vi "Tap_valuation.vi"(0 "1st_Col.":i32, 1 "1st_moveLog":i32[][](array[numeric]), 3 "1st_TotalP":i32, 5 "1st_TapN":dbl, 9 "2nd_TotalP":i32, 11 "2nd_moveLog":i32[][](array[numeric]), 12 "2nd Col.":i32, 13 "2nd_TapN":dbl, 14 "start Col.":i32) -> (4 "1st or 2nd":enum16{"1>2", "1=2", "1<2"}(ring), 6 "Out_TotalP":i32, 8 "Out_TapN":dbl, 10 "OutPut_moveLog":i32[][](array[numeric]), 15 "Out_ Col.":i32)   [LabVIEW 2016]
panel:
  out "Result":string
  out "1stmoveN":i32
  out "2ndmoveN":i32
  # "優先順位(1:1st, 2:2nd)\n① : TapN \n      ①-1 : 1<2 → 1\n      ①-2 : 1>2 → 2\n      ①-3 : 1=2 → ②へ\n② : start Col. dev\n      ②-1 : |1-s|<|2-s|→1\n      ②-2 : |1-s|>|2-s|→2\n      ③-3 : |1-s|=|2-s|→③\n③ : TotalP\n　　　③-1 : 1≦2 →1\n      ③-2 : 1>2 → 2\n　　　③-3 : 1=2 → ④\n④: moveLogの移動少なさ\n　　　④-1 : 1≦2 →1\n      ④-2 : 1>2 → 2\n　　　④-3 : 1=2 → ④"
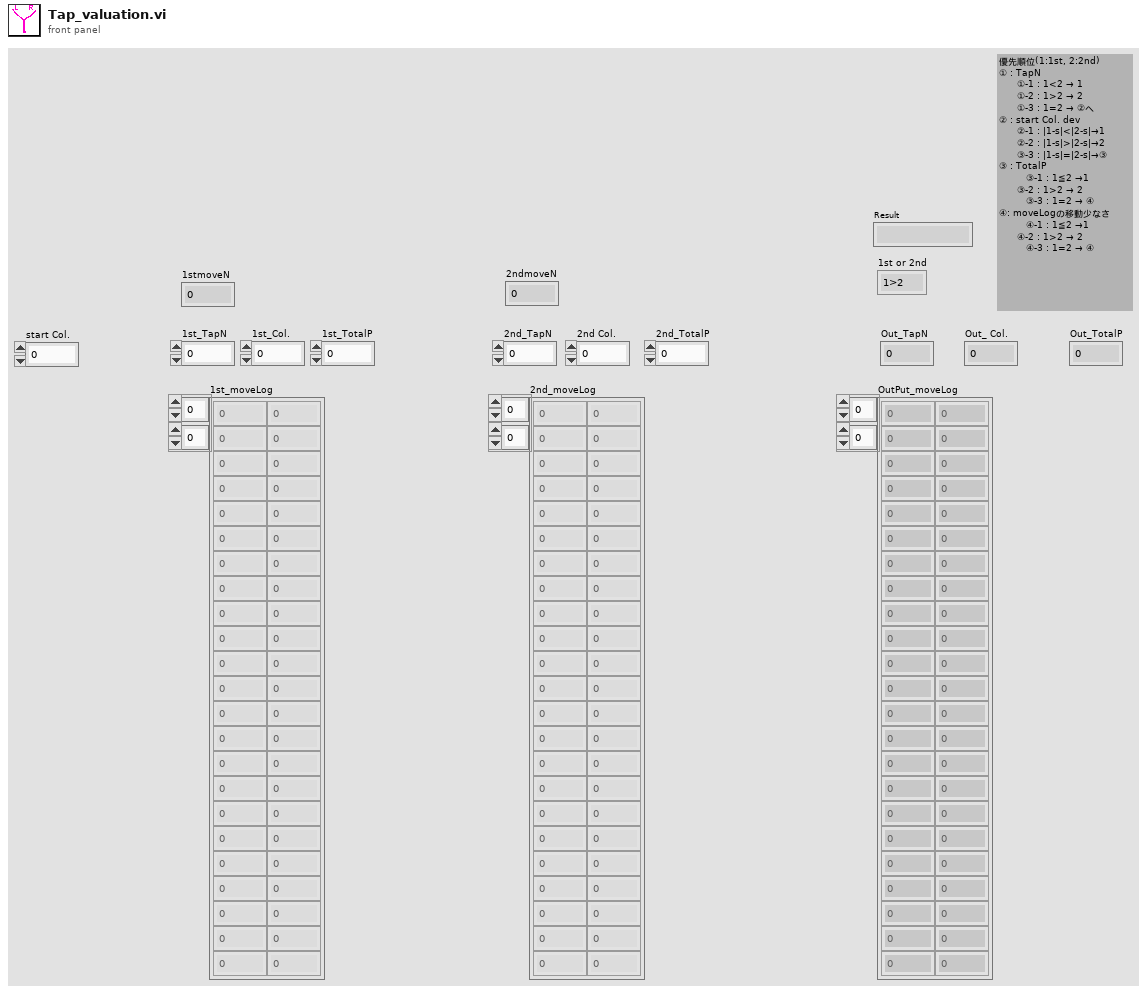
[diagram p1: front panel]
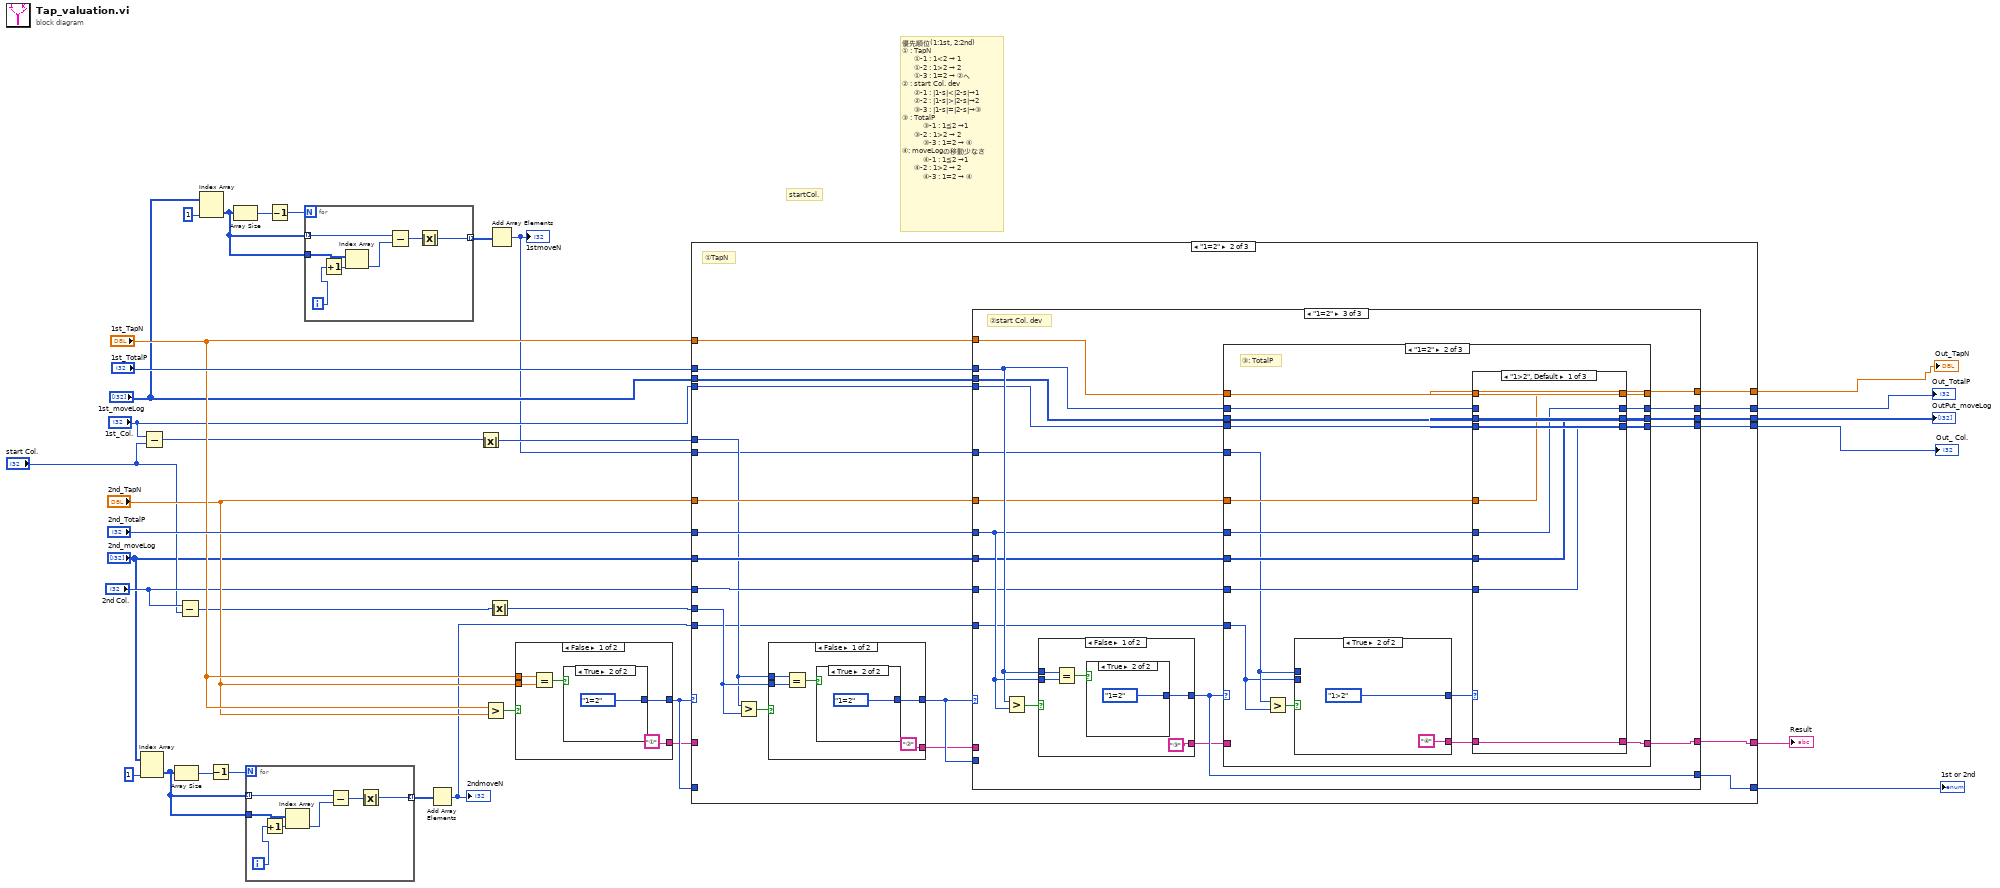
[diagram p0: block diagram]
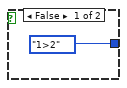
[diagram p2: hidden frame]
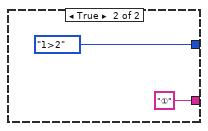
[diagram p3: hidden frame]
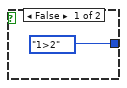
[diagram p5: hidden frame]
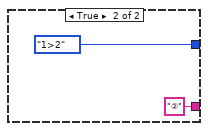
[diagram p6: hidden frame]
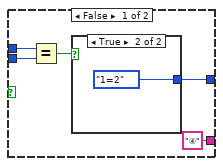
[diagram p12: hidden frame]
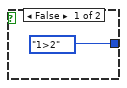
[diagram p13: hidden frame]
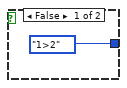
[diagram p15: hidden frame]
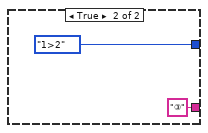
[diagram p16: hidden frame]
diagram:
  # "優先順位(1:1st, 2:2nd)\n① : TapN \n      ①-1 : 1<2 → 1\n      ①-2 : 1>2 → 2\n      ①-3 : 1=2 → ②へ\n② : start Col. dev\n      ②-1 : |1-s|<|2-s|→1\n      ②-2 : |1-s|>|2-s|→2\n      ③-3 : |1-s|=|2-s|→③\n③ : TotalP\n　　　③-1 : 1≦2 →1\n      ③-2 : 1>2 → 2\n　　　③-3 : 1=2 → ④\n④: moveLogの移動少なさ\n　　　④-1 : 1≦2 →1\n      ④-2 : 1>2 → 2\n　　　④-3 : 1=2 → ④"
  # "startCol."
  n1 = Index Array(array="2nd_moveLog", index (col)=1 ("無効な指標 （列）")) -> (element=w14:i32[])  [unwired: 1 in]
  n2 = Subtract(x="1st_Col.", y="start Col.") -> (x-y=w22:i32)
  n3 = Array Size(array=w14) -> (size(s)=w13:i32)
  n4 = Subtract(x="2nd Col.", y="start Col.") -> (x-y=w20:i32)
  n5 = Index Array(array="1st_moveLog", index (col)=1 ("無効な指標 （列）")) -> (element=w7:i32[])  [unwired: 1 in]
  n6 = Decrement(x=w13) -> (x-1=w12:i32)
  n7 = Array Size(array=w7) -> (size(s)=w8:i32)
  n8 = for {
    N: w12 -> [_]
    tunnel: w14 -> [w38] mode=indexing
    tunnel: w14 -> [w41]
    tunnel: [w35] -> w11 mode=indexing
    i -> [w39]
    n9 = Increment(x=w39) -> (x+1=w40:i32)
    n10 = Index Array(array=w41, index=w40) -> (element=w37:i32)
    n11 = Subtract(x=w38, y=w37) -> (x-y=w36:i32)
    n12 = Absolute Value(x=w36) -> (abs(x)=w35:i32)
  }
  n13 = Decrement(x=w8) -> (x-1=w9:i32)
  n14 = for {
    N: w9 -> [_]
    tunnel: w7 -> [w45] mode=indexing
    tunnel: w7 -> [w48]
    tunnel: [w42] -> w10 mode=indexing
    i -> [w46]
    n15 = Increment(x=w46) -> (x+1=w47:i32)
    n16 = Index Array(array=w48, index=w47) -> (element=w44:i32)
    n17 = Subtract(x=w45, y=w44) -> (x-y=w43:i32)
    n18 = Absolute Value(x=w43) -> (abs(x)=w42:i32)
  }
  n19 = Add Array Elements(numeric array=w11) -> (sum=w3:i32)
  "2ndmoveN" <- w3
  n20 = Absolute Value(x=w22) -> (abs(x)=w21:i32)
  n21 = Greater?(x="1st_TapN", y="2nd_TapN") -> (0:w28:bool)
  n22 = Absolute Value(x=w20) -> (abs(x)=w19:i32)
  n23 = Add Array Elements(numeric array=w10) -> (sum=w4:i32)
  "1stmoveN" <- w4
  n24 = case shown="False" w28 {
    tunnel: [w53 enum16{"1>2", "1=2", "1<2"}."1>2"] -> w18
    tunnel: "1st_TapN" -> [w52 _]
    tunnel: "2nd_TapN" -> [w51 _]
    tunnel: ["①" "①"] -> w2
    frame False {
      n25 = Equal?(x=w52, y=w51) -> (x = y?=w50:bool)
      n26 = case shown="True" w50 {
        tunnel: [enum16{"1>2", "1=2", "1<2"}."1>2" enum16{"1>2", "1=2", "1<2"}."1=2"] -> w53
        frame False {
        }
        frame True {
        }
      }
    }
    frame True {
    }
  }
  n27 = case shown="\"1=2\"" w18 {
    tunnel: "2nd_moveLog" -> [w61 w84 _]
    tunnel: "1st_moveLog" -> [_ w82 w190]
    tunnel: "2nd Col." -> [w60 w83 _]
    tunnel: "1st_Col." -> [_ w81 w188]
    tunnel: [w61 w79 w190] -> w32
    tunnel: "1st_TotalP" -> [_ w74 w189]
    tunnel: "2nd_TotalP" -> [w62 w73 _]
    tunnel: [w62 w80 w189] -> w31
    tunnel: [w60 w78 w188] -> w30
    tunnel: "2nd_TapN" -> [w63 w76 _]
    tunnel: "1st_TapN" -> [_ w75 w187]
    tunnel: [w63 w77 w187] -> w29
    tunnel: w21 -> [_ w70 _]
    tunnel: w19 -> [_ w71 _]
    tunnel: w18 -> [w59 _ w186]
    tunnel: [w59 w68 w186] -> w17
    tunnel: w4 -> [_ w67 _]
    tunnel: w3 -> [_ w66 _]
    tunnel: w2 -> [w58 _ w185]
    tunnel: [w58 w65 w185] -> w1
    frame "1>2", Default {
    }
    frame "1=2" {
      # "①TapN"
      n28 = Greater?(x=w70, y=w71) -> (0:w72:bool)
      n29 = case shown="False" w72 {
        tunnel: [w89 enum16{"1>2", "1=2", "1<2"}."1>2"] -> w69
        tunnel: w70 -> [w88 _]
        tunnel: w71 -> [w87 _]
        tunnel: ["②" "②"] -> w64
        frame False {
          n30 = Equal?(x=w88, y=w87) -> (x = y?=w86:bool)
          n31 = case shown="True" w86 {
            tunnel: [enum16{"1>2", "1=2", "1<2"}."1>2" enum16{"1>2", "1=2", "1<2"}."1=2"] -> w89
            frame False {
            }
            frame True {
            }
          }
        }
        frame True {
        }
      }
      n32 = case shown="\"1=2\"" w69 {
        tunnel: [w98 w105 w119] -> w80
        tunnel: w73 -> [w98 _ w113]
        tunnel: w84 -> [w97 _ w112]
        tunnel: [w97 w104 w118] -> w79
        tunnel: [w96 w103 w116] -> w78
        tunnel: w83 -> [w96 _ w111]
        tunnel: w74 -> [_ w105 w120]
        tunnel: w82 -> [_ w104 w117]
        tunnel: w81 -> [_ w103 w115]
        tunnel: w75 -> [_ w102 w121]
        tunnel: [w99 w102 w122] -> w77
        tunnel: w76 -> [w99 _ w114]
        tunnel: w69 -> [w95 w101 _]
        tunnel: [w95 w101 w110] -> w68
        tunnel: w67 -> [_ _ w109]
        tunnel: w66 -> [_ _ w108]
        tunnel: [w94 w100 w107] -> w65
        tunnel: w64 -> [w94 w100 _]
        frame "1>2", Default {
        }
        frame "1<2" {
        }
        frame "1=2" {
          # "②start Col. dev"
          n33 = Greater?(x=w120, y=w113) -> (0:w123:bool)
          n34 = case shown="False" w123 {
            tunnel: [w180 enum16{"1>2", "1=2", "1<2"}."1>2"] -> w110
            tunnel: w120 -> [w179 _]
            tunnel: w113 -> [w178 _]
            tunnel: ["③" "③"] -> w106
            frame False {
              n35 = Equal?(x=w179, y=w178) -> (x = y?=w177:bool)
              n36 = case shown="True" w177 {
                tunnel: [enum16{"1>2", "1=2", "1<2"}."1>2" enum16{"1>2", "1=2", "1<2"}."1=2"] -> w180
                frame False {
                }
                frame True {
                }
              }
            }
            frame True {
            }
          }
          n37 = case shown="\"1=2\"" w110 {
            tunnel: [w128 w144 w175] -> w122
            tunnel: w121 -> [_ w143 w175]
            tunnel: w120 -> [_ w141 w174]
            tunnel: [w127 w142 w174] -> w119
            tunnel: [w126 w140 w173] -> w118
            tunnel: w117 -> [_ w139 w173]
            tunnel: w115 -> [_ w137 w172]
            tunnel: [w125 w138 w172] -> w116
            tunnel: w114 -> [w128 w136 _]
            tunnel: w113 -> [w127 w135 _]
            tunnel: w112 -> [w126 w134 _]
            tunnel: w111 -> [w125 w133 _]
            tunnel: w109 -> [_ w132 _]
            tunnel: w108 -> [_ w131 _]
            tunnel: [w124 w130 w171] -> w107
            tunnel: w106 -> [w124 _ w171]
            frame "1>2", Default {
            }
            frame "1=2" {
              # "③: TotalP"
              n38 = Greater?(x=w132, y=w131) -> (0:w146:bool)
              n39 = case shown="True" w146 {
                tunnel: [w166 enum16{"1>2", "1=2", "1<2"}."1>2"] -> w145
                tunnel: w132 -> [w165 _]
                tunnel: w131 -> [w164 _]
                tunnel: ["④" "④"] -> w129
                frame False {
                  n40 = Equal?(x=w165, y=w164) -> (x = y?=w163:bool)
                  n41 = case shown="True" w163 {
                    tunnel: [enum16{"1>2", "1=2", "1<2"}."1>2" enum16{"1>2", "1=2", "1<2"}."1=2"] -> w166
                    frame False {
                    }
                    frame True {
                    }
                  }
                }
                frame True {
                }
              }
              n42 = case shown="\"1>2\", Default" w145 {
                tunnel: [w151 w156 w161] -> w144
                tunnel: w143 -> [_ w156 w161]
                tunnel: [w150 w155 w160] -> w142
                tunnel: w141 -> [_ w155 w160]
                tunnel: [w149 w154 w159] -> w140
                tunnel: w139 -> [_ w154 w159]
                tunnel: [w148 w153 w158] -> w138
                tunnel: w137 -> [_ w153 w158]
                tunnel: w136 -> [w151 _ _]
                tunnel: w135 -> [w150 _ _]
                tunnel: w134 -> [w149 _ _]
                tunnel: w133 -> [w148 _ _]
                tunnel: [w147 w152 w157] -> w130
                tunnel: w129 -> [w147 w152 w157]
                frame "1>2", Default {
                }
                frame "1<2" {
                }
                frame "1=2" {
                }
              }
            }
            frame "1<2" {
            }
          }
        }
      }
    }
    frame "1<2" {
      # "Right"
    }
  }
  "OutPut_moveLog" <- w32
  "Out_TotalP" <- w31
  "Out_ Col." <- w30
  "Out_TapN" <- w29
  "1st or 2nd" <- w17
  "Result" <- w1
